vi "Monitor Active Project.vi"(10 "Active Project Changed":refnum<user-event>) -> ()   [LabVIEW 2017, in "Test Explorer.lvlib"]
doc: "Generates a user event when the active project in the current application instance changed. This VI keeps running until the specified user event is destroyed."
uses:
  Test Explorer.lvlib
  b8ae5672-8134-400f-a408-93b2af799a79.vi
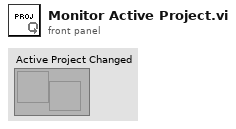
[diagram p1: front panel]
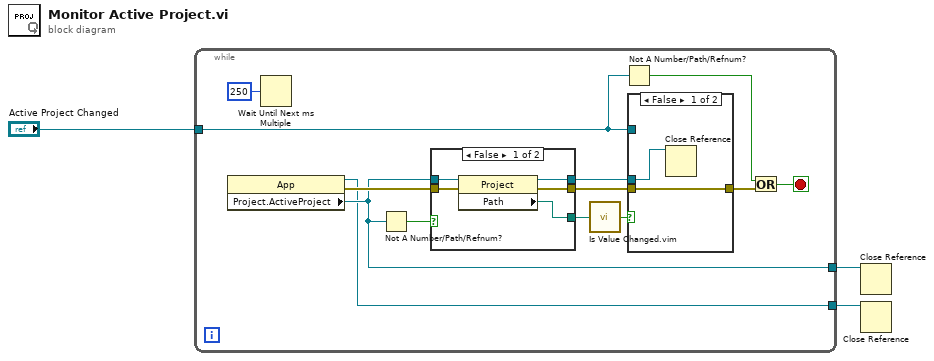
[diagram p0: block diagram]
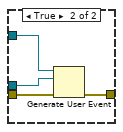
[diagram p3: hidden frame]
diagram:
  n1 = while {
    tunnel: "Active Project Changed" -> [w8]
    tunnel: [w5] -> w2
    tunnel: [w4] -> w1
    stop <- w9 stop-if-true
    n2 = property class="App"() -> (reference out=w4:refnum<vi>, error out=w16:errorcluster, "Project.ActiveProject"=w5:refnum<vi>)  [unwired: 2 in]
    n3 = Wait Until Next ms Multiple(millisecond multiple=u32 250) -> ()  [unwired: 1 out]
    n4 = Not A Number/Path/Refnum?(number/path/refnum=w5) -> (NaN/Path/Refnum?=w10:bool)
    n5 = case shown="False" w10 {
      tunnel: w16 -> [w21 w22]
      tunnel: w5 -> [w20 w23]
      tunnel: [w19 _] -> w15
      tunnel: [w18 w23] -> w13
      tunnel: [w17 w22] -> w12
      frame False {
        n6 = property class="Project"(reference=w20, error in=w21) -> (reference out=w18:refnum<vi>, error out=w17:errorcluster, "Path"=w19:path)
      }
      frame True {
      }
    }
    n7 = call "Is Value Changed.vim"("value"=w15) -> ("changed or first call?"=w14:bool)
    n8 = Not A Number/Path/Refnum?(number/path/refnum=w8) -> (NaN/Path/Refnum?=w7:bool)
    n9 = case shown="False" w14 {
      tunnel: w8 -> [_ w29]
      tunnel: w13 -> [w24 w28]
      tunnel: w12 -> [w25 w27]
      tunnel: [w25 w26] -> w6
      frame False {
        n10 = Close Reference(reference=w24) -> ()  [unwired: 1 in, 1 out]
      }
      frame True {
        n11 = Generate User Event(user event=w29, event data cluster=w28, error in=w27) -> (error out=w26:errorcluster)  [unwired: 1 in, 1 out]
      }
    }
    n12 = Or(x=w7, y=w6) -> (x .or. y?=w9:bool)
  }
  n13 = Close Reference(reference=w2) -> ()  [unwired: 1 in, 1 out]
  n14 = Close Reference(reference=w1) -> ()  [unwired: 1 in, 1 out]
